vi "Motor control FPGA with encoder reading.vi"() -> ()   [LabVIEW 2013]
uses:
  <vilib>/eio/EIONode/EIONode.xnode
  <vilib>/rvi/eio/common/nirviEmuTemplateMethod_errors.vi
panel:
  out "Pulses":i16
  out "Degree (absolute)":i16
  out "Degree (relative)":i16
  out "Tours":i16
  in  "Position Reset":bool
  out "Position (Counts)":i64
  in  "Velocity Interval (uSec)":u32
  out "Acceleration (Counts/Interval)":i64
  out "Velocity (Counts/Interval)":i64
  in  "Cluster":T1
  in  "Direction":bool
  in  "Enable":bool
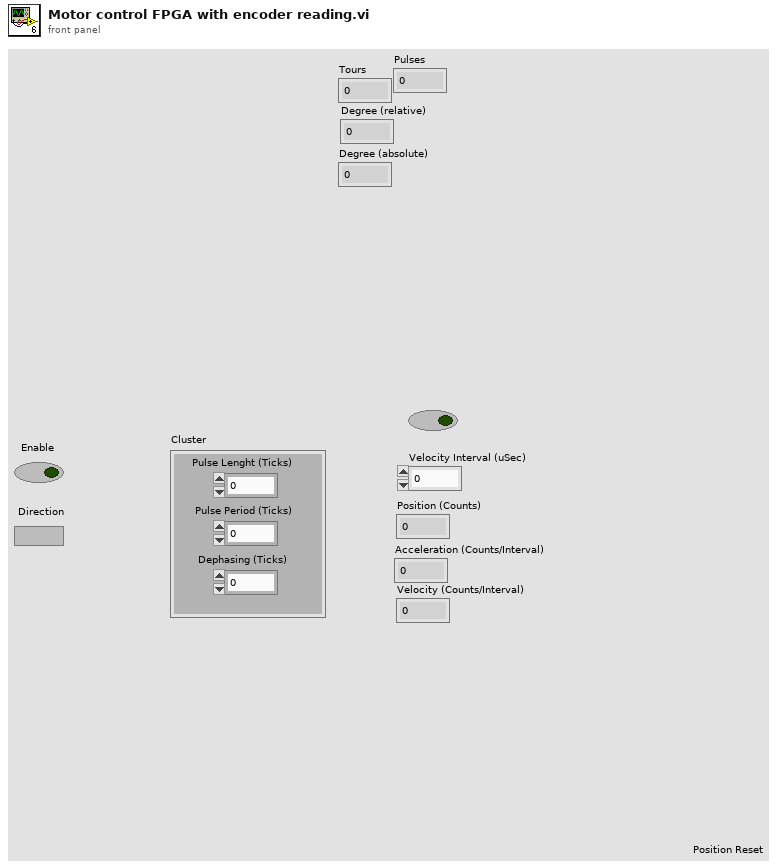
[diagram p1: front panel]
types:
  T1 = cluster{"Pulse Lenght (Ticks)":i16, "Pulse Period (Ticks)":i16, "Dephasing (Ticks)":i16}
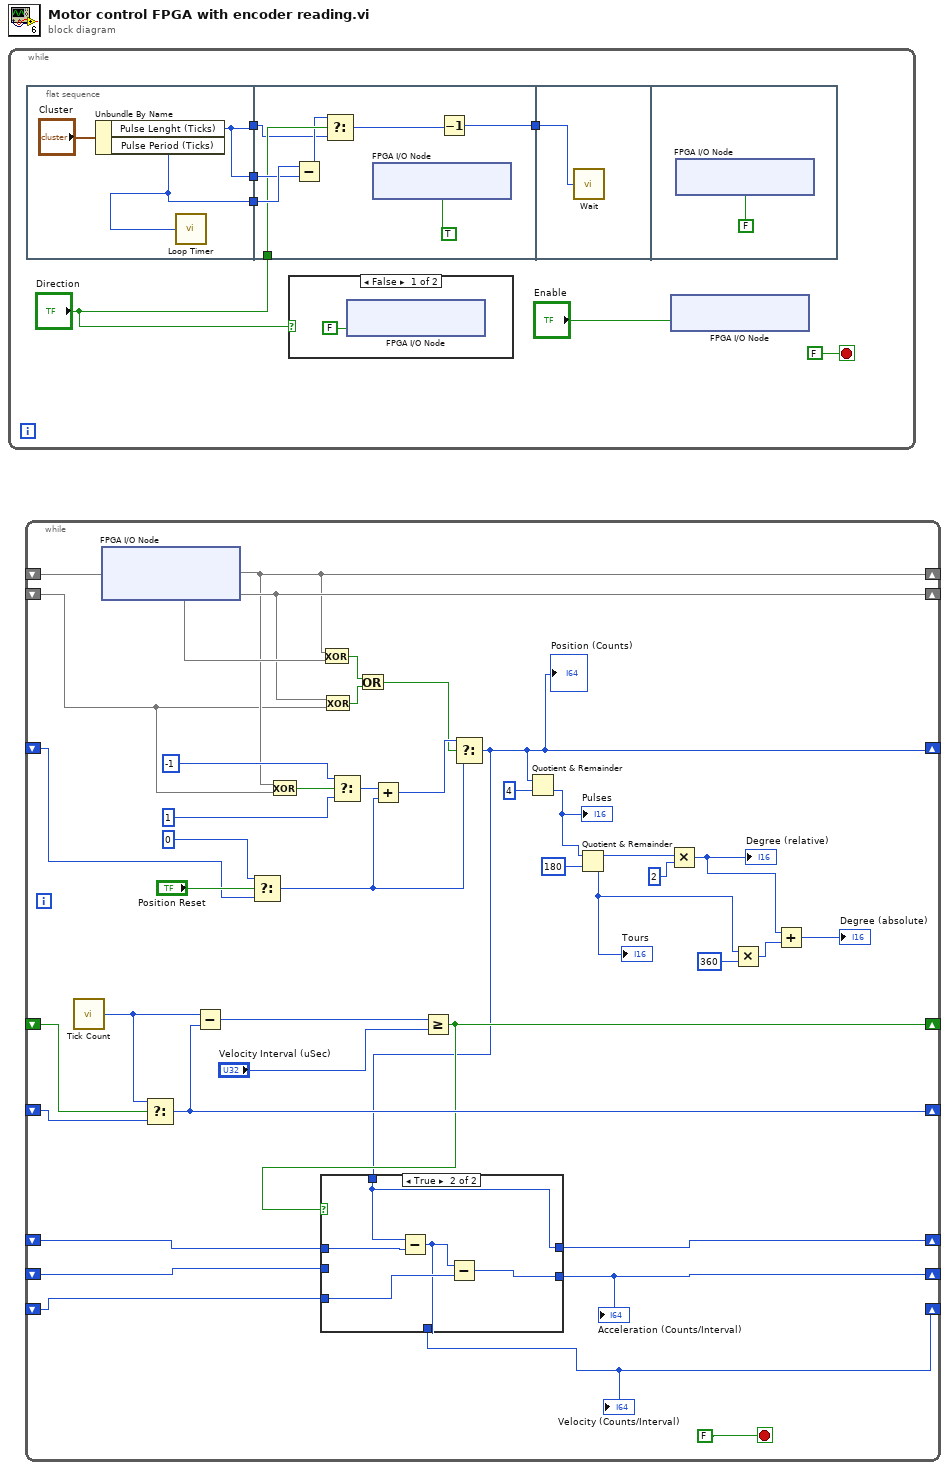
[diagram p0: block diagram]
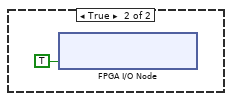
[diagram p3: hidden frame]
diagram:
  n1 = while {
    stop <- FALSE stop-if-true
    n2 = flat-sequence {
      tunnel: [w10] -> w7
      tunnel: [w11] -> w4
      tunnel: [w10] -> w3
      tunnel: w7 -> [w13]
      tunnel: [w19] -> w6
      tunnel: w4 -> [w17]
      tunnel: w3 -> [w16]
      tunnel: "Direction" -> [w15]
      tunnel: w6 -> [w21]
      frame #0 {
        n3 = Unbundle By Name("Cluster") -> ("Pulse Lenght (Ticks)"=w10:i16, "Pulse Period (Ticks)"=w11:i16)
        n4 = call "Loop Timer"("Count(Ticks)"=w11) -> ()  [unwired: 1 out]
      }
      frame #1 {
        n5 = Subtract(x=w17, y=w16) -> (x-y=w14:i16)
        n6 = Select(t=w14, s=w15, f=w13) -> (s? t:f=w18:i16)
        n7 = xnode "FPGA I/O Node"("ConnectorC/DIO3"=TRUE ("ConnectorC/DIO7")) -> ()  [unwired: 1 in, 1 out]
        n8 = Decrement(x=w18) -> (x-1=w19:i16)
      }
      frame #2 {
        n9 = call "Wait"("Count(Ticks)"=w21) -> ()  [unwired: 1 out]
      }
      frame #3 {
        n10 = xnode "FPGA I/O Node"("ConnectorC/DIO3"=FALSE ("ConnectorC/DIO7")) -> ()  [unwired: 1 in, 1 out]
      }
    }
    n11 = case shown="False" "Direction" {
      frame False {
        n12 = xnode "FPGA I/O Node"("ConnectorC/DIO7"=FALSE) -> ()  [unwired: 1 in, 1 out]
      }
      frame True {
        n13 = xnode "FPGA I/O Node"("ConnectorC/DIO7"=TRUE) -> ()  [unwired: 1 in, 1 out]
      }
    }
    n14 = xnode "FPGA I/O Node"("ConnectorA/DIO0"="Enable") -> ()  [unwired: 1 in, 1 out]
  }
  n15 = while {
    shift-right: [w27] -> _
    shift-left: _ -> [w63]
    shift-right: [w40] -> _
    shift-left: _ -> [w26]
    shift-right: [w23] -> _
    shift-left: _ -> [w36]
    shift-right: [w48] -> _
    shift-left: _ -> [w51]
    shift-right: [w49] -> _
    shift-left: _ -> [w50]
    shift-right: [w46] -> _
    shift-left: _ -> [w47]
    shift-right: [w45] -> _
    shift-left: _ -> [w42]
    shift-right: [w43] -> _
    shift-left: _ -> [w44]
    stop <- FALSE stop-if-true
    n16 = call "Tick Count"() -> ("Tick Count(Ticks)"=w53:u32)
    n17 = xnode "FPGA I/O Node"() -> ("ConnectorA/DIO6"=w27, "ConnectorA/DIO7"=w40)  [unwired: 2 in, 2 out]
    n18 = Select(t=w53, s=w51, f=w50) -> (s? t:f=w49:u32)
    n19 = Subtract(x=w53, y=w49) -> (x-y=w54:u32)
    n20 = Select(t=i16 0, s="Position Reset", f=w36) -> (s? t:f=w55:i16)
    n21 = Exclusive Or(1:w26, 2:w27) -> (0:w39:bool)
    n22 = Exclusive Or(1:w63, 2:w27) -> (0:w62:bool)
    n23 = Exclusive Or(1:w26, 2:w40) -> (0:w61:bool)
    n24 = Select(t=i16 -1, s=w39, f=i16 1) -> (s? t:f=w57:i16)
    n25 = Or(x=w62, y=w61) -> (x .or. y?=w37:bool)
    n26 = Add(x=w57, y=w55) -> (x+y=w56:i16)
    n27 = Greater Or Equal?(x=w54, y="Velocity Interval (uSec)") -> (x >= y?=w48:bool)
    n28 = Select(t=w56, s=w37, f=w55) -> (s? t:f=w23:i16)
    "Position (Counts)" <- w23
    n29 = case shown="True" w48 {
      tunnel: w47 -> [w66 w71]
      tunnel: w23 -> [_ w70]
      tunnel: [w66 w70] -> w46
      tunnel: [w65 w69] -> w45
      tunnel: w44 -> [w64 w68]
      tunnel: [w64 w67] -> w43
      tunnel: w42 -> [w65 _]
      frame False {
      }
      frame True {
        n30 = Subtract(x=w70, y=w71) -> (x-y=w67:i16)
        n31 = Subtract(x=w67, y=w68) -> (x-y=w69:i16)
      }
    }
    "Acceleration (Counts/Interval)" <- w45
    "Velocity (Counts/Interval)" <- w43
    n32 = Quotient & Remainder(x=w23, y=i16 4) -> (floor(x/y)=w24:i16)  [unwired: 1 out]
    "Pulses" <- w24
    n33 = Quotient & Remainder(x=w24, y=i16 180) -> (x-y*floor(x/y)=w34:i16, floor(x/y)=w28:i16)
    "Tours" <- w28
    n34 = Multiply(x=w34, y=i16 2) -> (x*y=w31:i16)
    "Degree (relative)" <- w31
    n35 = Multiply(x=w28, y=i16 360) -> (x*y=w30:i16)
    n36 = Add(x=w31, y=w30) -> (x+y=→"Degree (absolute)":i16)
  }
